vi "temseq_new2.vi"() -> ()   [LabVIEW 2015]
uses:
  BERTTA.dll
panel:
  out "start_time":dbl
  out "Waveform Chart":dynamicdata(graph)
  in  "port":i32=9
  out "params":dbl[](array[numeric])
  in  "TimeParams":i32[](array[numeric])=[1, 1, 1, 1, 1]
  in  "SeqParams":dbl[](array[numeric])=[20.0, 35.0, 45.0, 20.0, 20.0, 35.0, 45.0, 20.0, 20.0, 20.0, 20.0, 20.0, 20.0, 20.0, 20.0, 40.0, 2.0, 1.0]
  out "Tr":dbl
  in  "Tr_orTj":i32
  in  "shutdown":i32
  in  "pause":i32
  in  "master":i32
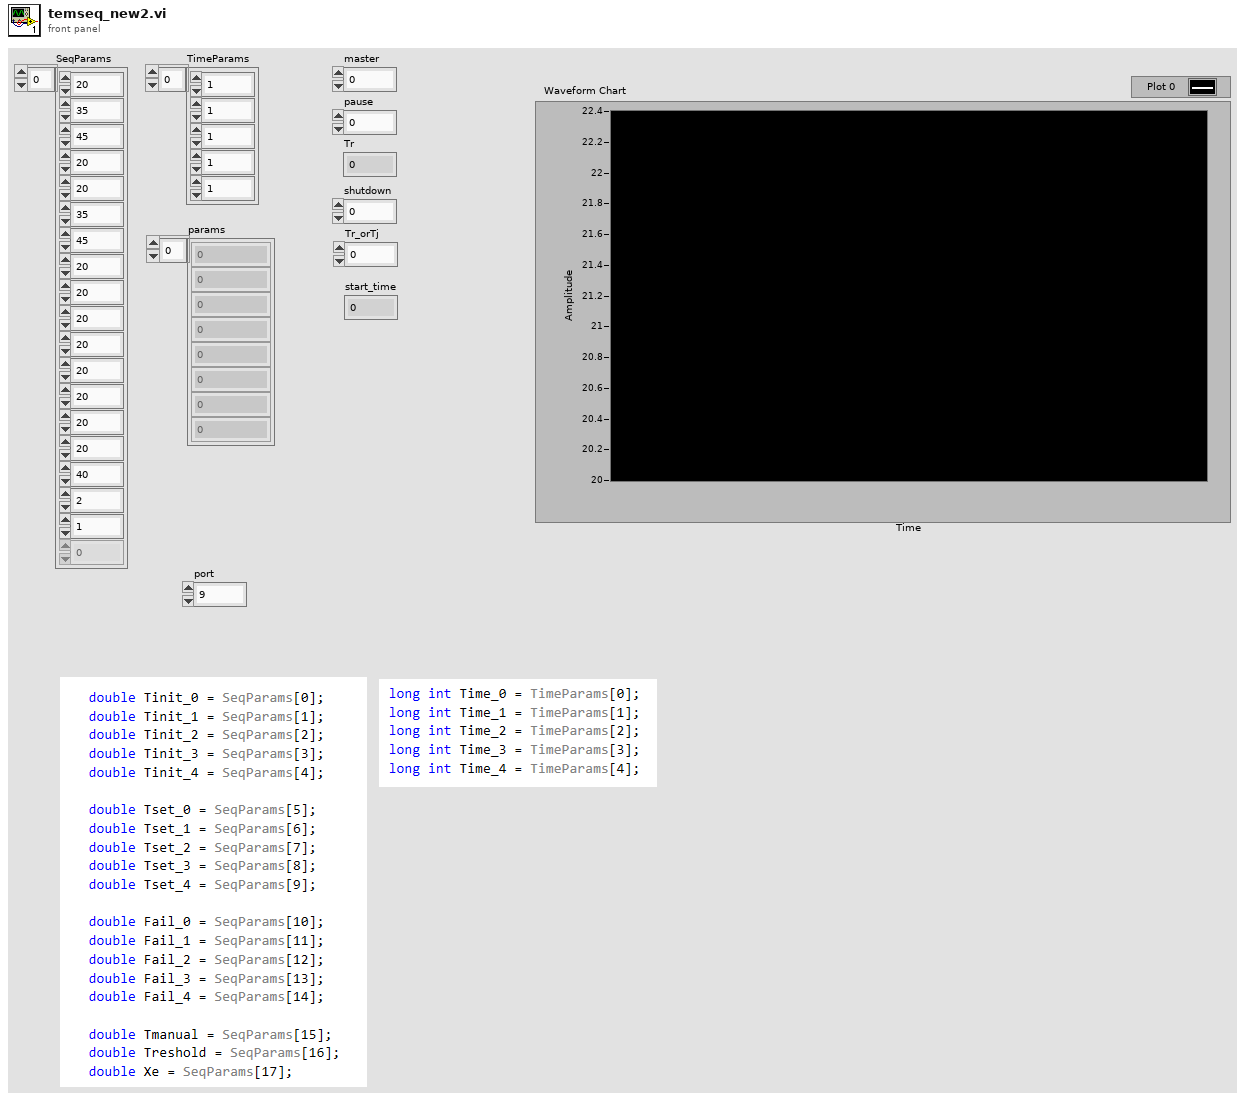
[diagram p1: front panel]
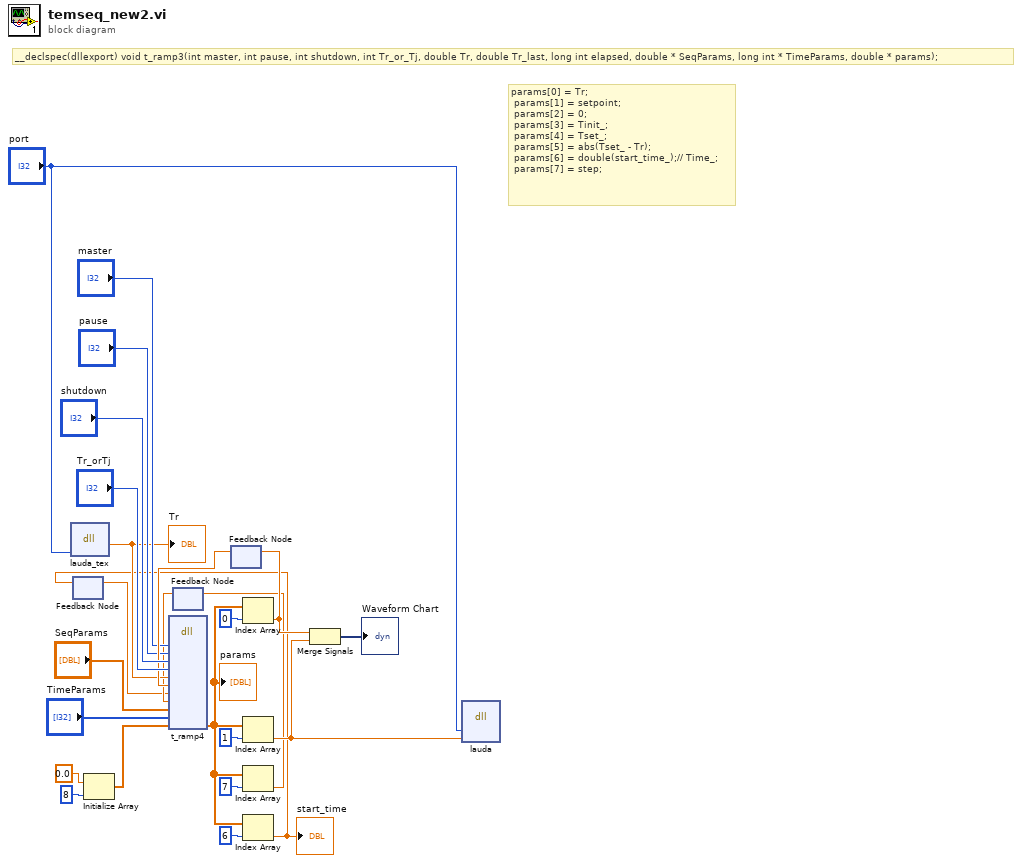
[diagram p0: block diagram]
diagram:
  # "params[0] = Tr;\n\tparams[1] = setpoint;\n\tparams[2] = 0;\n\tparams[3] = Tinit_;\n\tparams[4] = Tset_;\n\tparams[5] = abs(Tset_ - Tr);\n\tparams[6] = double(start_time_);// Time_;\n\tparams[7] = step;"
  # "__declspec(dllexport) void t_ramp3(int master, int pause, int shutdown, int Tr_or_Tj, double Tr, double Tr_last, long int elapsed, double * SeqParams, long int * TimeParams, double * params);"
  n1 = dll-call lib="C:/Users/shresplab/OneDrive - Kemira Oyj/Documents/Visual Studio 2017/Projects/Bertta/BERTTA/x64/Debug/BERTTA.dll" fn="lauda_tex"("port"="port") -> ("return type"=w11:dbl)  [unwired: 4 in, 2 out]
  "Tr" <- w11
  n2 = feedback #1() -> (w1:dbl)  [unwired: 1 in]
  n3 = Initialize Array(0.0 ("element"), 8 ("dimension size")) -> (w18:dbl[])
  n4 = feedback #2() -> (w5:dbl)  [unwired: 1 in]
  n5 = feedback #3() -> (w16:dbl)  [unwired: 1 in]
  n6 = dll-call lib="C:/Users/shresplab/OneDrive - Kemira Oyj/Documents/Visual Studio 2017/Projects/Bertta/BERTTA/x64/Debug/BERTTA.dll" fn="t_ramp4"("master"="master", "pause"="pause", "shutdown"="shutdown", "Tr_orTj"="Tr_orTj", "Tr"=w11, "Tr_last"=w16, "start_time"=w1, "step_previous"=w5, "SeqParams"="SeqParams", "TimeParams"="TimeParams", "params"=w18) -> ("params"=w3:dbl[])  [unwired: 14 in, 2 out]
  "params" <- w3
  n7 = Index Array(array=w3, index=0) -> (element=w10:dbl)
  n8 = feedback-in #3(w10) -> ()
  n9 = Index Array(array=w3, index=1) -> (element=w9:dbl)
  n10 = Index Array(array=w3, index=7) -> (element=w6:dbl)
  n11 = feedback-in #2(w6) -> ()
  n12 = Index Array(array=w3, index=6) -> (element=w2:dbl)
  "start_time" <- w2
  n13 = feedback-in #1(w2) -> ()
  n14 = Merge Signals(w10, w9) -> (→"Waveform Chart":dynamicdata)
  n15 = dll-call lib="C:/Users/shresplab/OneDrive - Kemira Oyj/Documents/Visual Studio 2017/Projects/Bertta/BERTTA/x64/Debug/BERTTA.dll" fn="lauda"("port"="port", "set_temp"=w9) -> ()  [unwired: 6 in, 2 out]
